vi "Gear.vi"(10 "Actuate Gear":bool) -> ()   [LabVIEW 2016]
uses:
  <vilib>/Rock Robotics/WPI/Solenoid/WPI_SolenoidValue.ctl
  <vilib>/Rock Robotics/WPI/Solenoid/WPI_SolenoidSetEnum.vi
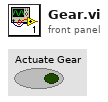
[diagram p1: front panel]
types:
  T1 = typedef "WPI_SolenoidValue.ctl" = enum16{"Off", "On", "Forward", "Reverse"}
  T2 = typedef "WPI_SolenoidDevRef.ctl" = cluster{"DevStatus":errorcluster, "Pneumatics Control Module":u8, "Forward Solenoid Channel":T3, "Reverse Solenoid Channel":T3}
  T3 = typedef "WPI_SolenoidChannel.ctl" = enum8{"Solenoid 0", "Solenoid 1", "Solenoid 2", "Solenoid 3", "Solenoid 4", "Solenoid 5", "Solenoid 6", "Solenoid 7", "Invalid"}
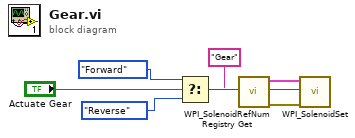
[diagram p0: block diagram]
diagram:
  n1 = Select(t=WPI_SolenoidValue."Forward" ("Value"), s="Actuate Gear", f=WPI_SolenoidValue."Reverse" ("Value")) -> (s? t:f=w5:T1)
  n2 = call <vilib>:"WPI_SolenoidRefNum Registry Get.vi"("refnum name"="Gear") -> ("error out"=w6:errorcluster, "SolenoidDevRef"=w7:T2)  [unwired: 9 in]
  n3 = call-poly <vilib>:"WPI_SolenoidSet.vi"("error in (no error)"=w6, "Value"=w5, "SolenoidDevRef"=w7) -> ()  [unwired: 7 in, 2 out]
